vi "svc_Check for Resampled Signal Continuity (no state).vi"(0 "even angle signal":T5 {"even angle signal" format="%.2f"; "dr" format="%.2f"; "r0" format="%.2f"}, 1 "even angle channel info":T1={"channel name"="", "description"="", " channel info"={"sensor sensitivity"=1000.0, "engineering units"=1, "dB reference"=1.0, "custom label"="EU", "weighting filter"=0, "pregain"=0.0}} {"channel info"."pregain" format="%.2f"; "channel info"."weighting filter" items=["Linear", "A-weighting", "B-weighting", "C-weighting", "ITU-R 468-4", "Dolby", "CCITT", "C-message", "Wb", "Wc", "Wd", "We", "Wf", "Wh", "Wj", "Wk", "Wm", "AES17 20 kHz lowpass", "AES17 40 kHz lowpass", "AES17 20 kHz highpass", "AES17 40 kHz highpass"]; "channel info"."dB reference" format="%^.1e"; "channel info"."engineering units" items=["custom..."=0, "V"=1, "A"=21, "C"=30, "pC"=31, "s"=32, "-"=29, "Pa"=2, "N"=20, "g"=3, "m/s^2"=4, "m/s"=5, "m"=6, "mm/s"=12, "mm"=13, "micron/s"=14, "micron"=15, "in/s^2"=7, "in/s"=8, "in"=9, "mil/s"=10, "mil"=11, "rad/s^2"=16, "rad/s"=17, "rad"=18, "deg/s^2"=26, "deg/s"=27, "deg"=28, "RPM"=22, "cycle/s^2"=23, "Hz"=24, "cycle"=25, "strain"=19]; "channel info"."sensor sensitivity" format="%#_5f"}, 2 "parameter controls":T6, 5 "error in (no error)":errorcluster, 6 "reset":bool, 7 "expected even angle channel info":T1={"channel name"="", "description"="", " channel info"={"sensor sensitivity"=1000.0, "engineering units"=1, "dB reference"=1.0, "custom label"="EU", "weighting filter"=0, "pregain"=0.0}} {"channel info"."pregain" format="%.2f"; "channel info"."weighting filter" items=["Linear", "A-weighting", "B-weighting", "C-weighting", "ITU-R 468-4", "Dolby", "CCITT", "C-message", "Wb", "Wc", "Wd", "We", "Wf", "Wh", "Wj", "Wk", "Wm", "AES17 20 kHz lowpass", "AES17 40 kHz lowpass", "AES17 20 kHz highpass", "AES17 40 kHz highpass"]; "channel info"."dB reference" format="%^.1e"; "channel info"."engineering units" items=["custom..."=0, "V"=1, "A"=21, "C"=30, "pC"=31, "s"=32, "-"=29, "Pa"=2, "N"=20, "g"=3, "m/s^2"=4, "m/s"=5, "m"=6, "mm/s"=12, "mm"=13, "micron/s"=14, "micron"=15, "in/s^2"=7, "in/s"=8, "in"=9, "mil/s"=10, "mil"=11, "rad/s^2"=16, "rad/s"=17, "rad"=18, "deg/s^2"=26, "deg/s"=27, "deg"=28, "RPM"=22, "cycle/s^2"=23, "Hz"=24, "cycle"=25, "strain"=19]; "channel info"."sensor sensitivity" format="%#_5f"}, 9 "expected signal parameters":cluster{"r0":dbl, "dr":dbl, "array length":i32}) -> (11 "next expected signal parameters":cluster{"r0":dbl, "dr":dbl, "array length":i32}, 13 "even angle channel info":T1={"channel name"="", "description"="", " channel info"={"sensor sensitivity"=1000.0, "engineering units"=1, "dB reference"=1.0, "custom label"="EU", "weighting filter"=0, "pregain"=0.0}} {"channel info"."pregain" format="%.2f"; "channel info"."weighting filter" items=["Linear", "A-weighting", "B-weighting", "C-weighting", "ITU-R 468-4", "Dolby", "CCITT", "C-message", "Wb", "Wc", "Wd", "We", "Wf", "Wh", "Wj", "Wk", "Wm", "AES17 20 kHz lowpass", "AES17 40 kHz lowpass", "AES17 20 kHz highpass", "AES17 40 kHz highpass"]; "channel info"."dB reference" format="%^.1e"; "channel info"."engineering units" items=["custom..."=0, "V"=1, "A"=21, "C"=30, "pC"=31, "s"=32, "-"=29, "Pa"=2, "N"=20, "g"=3, "m/s^2"=4, "m/s"=5, "m"=6, "mm/s"=12, "mm"=13, "micron/s"=14, "micron"=15, "in/s^2"=7, "in/s"=8, "in"=9, "mil/s"=10, "mil"=11, "rad/s^2"=16, "rad/s"=17, "rad"=18, "deg/s^2"=26, "deg/s"=27, "deg"=28, "RPM"=22, "cycle/s^2"=23, "Hz"=24, "cycle"=25, "strain"=19]; "channel info"."sensor sensitivity" format="%#_5f"}, 14 "even angle signal":T5 {"even angle signal" format="%.2f"; "dr" format="%.2f"; "r0" format="%.2f"}, 15 "waveform parameter changed":bool, 16 "dt":dbl, 17 "array length":i32, 19 "error out":errorcluster)   [LabVIEW 2017]
uses:
  <vilib>/addons/_NISVFA/_Shared subVIs/Controls/svc_Resampled Channel Info.ctl
  <vilib>/addons/_NISVFA/_Shared subVIs/Controls/svc_Channel Info.ctl
  <vilib>/addons/_NISVFA/_Shared subVIs/Controls/svc_Engineering Units Text Ring.ctl
  <vilib>/addons/_NISVFA/_Shared subVIs/Controls/svc_Weighting Filter Text Ring.ctl
panel:
  in  "exact comparison for dr?":bool=TRUE
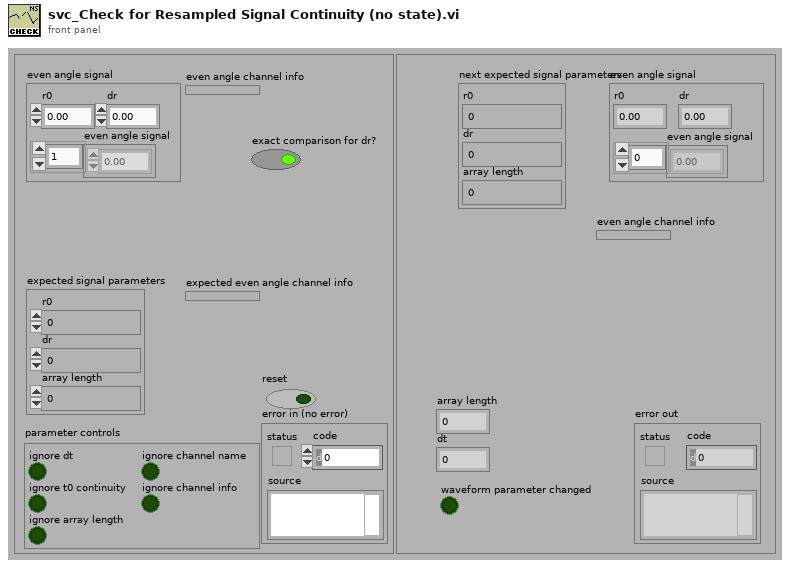
[diagram p1: front panel]
types:
  T1 = typedef "svc_Resampled Channel Info.ctl" = cluster{"channel name":string, "description":string, " channel info":T2}
  T2 = typedef "svc_Channel Info.ctl" = cluster{"sensor sensitivity":dbl, "engineering units":T3, "dB reference":dbl, "custom label":string, "weighting filter":T4, "pregain":dbl}
  T3 = typedef "svc_Engineering Units Text Ring.ctl" = u16
  T4 = typedef "svc_Weighting Filter Text Ring.ctl" = u16
  T5 = cluster{"r0":dbl, "dr":dbl, "even angle signal":dbl[]}
  T6 = cluster{"ignore dt":bool, "ignore t0 continuity":bool, "ignore array length":bool, "ignore channel info":bool, "ignore channel name":bool}
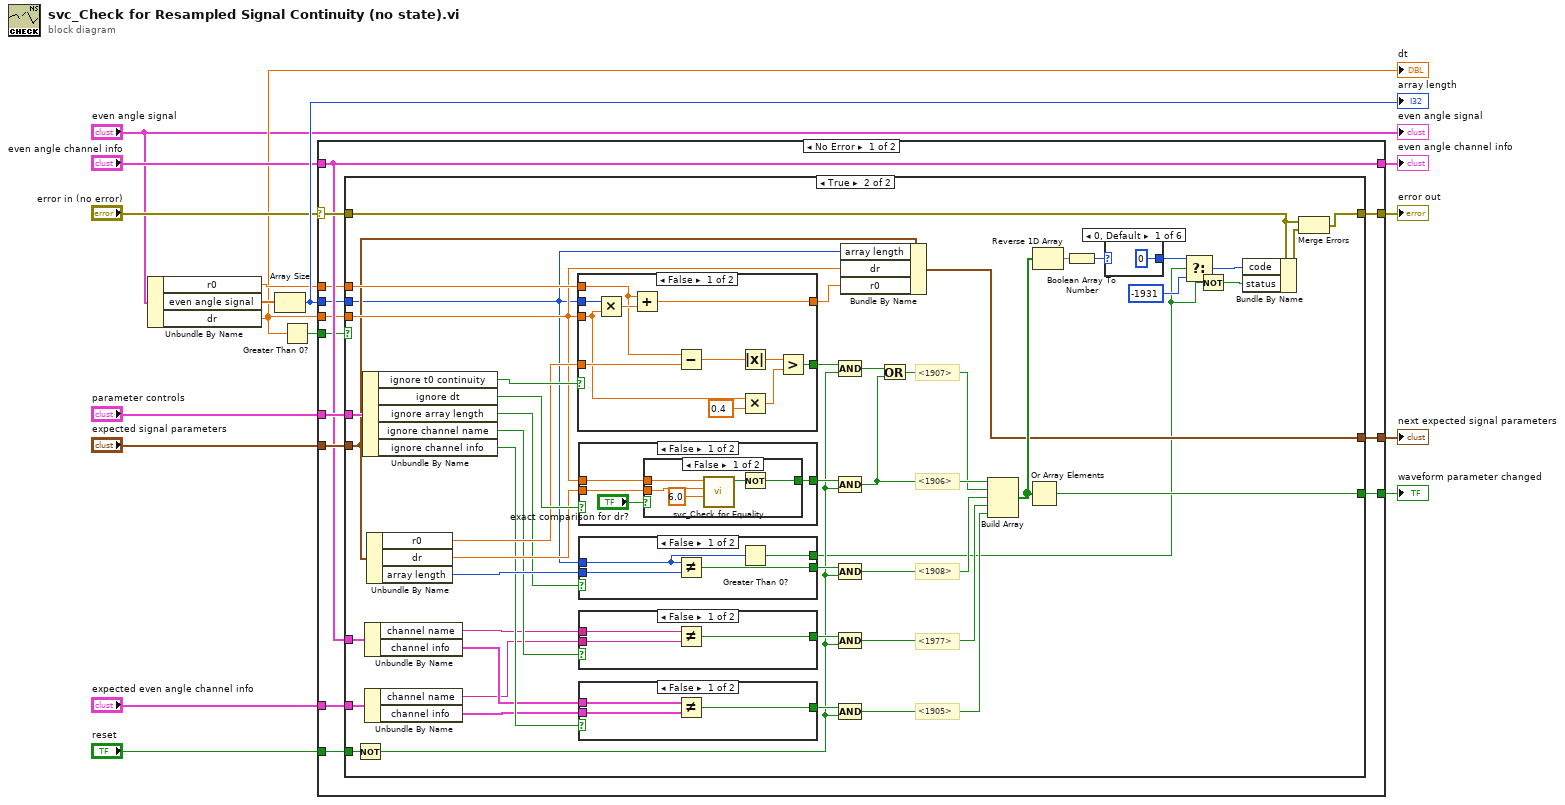
[diagram p0: block diagram]
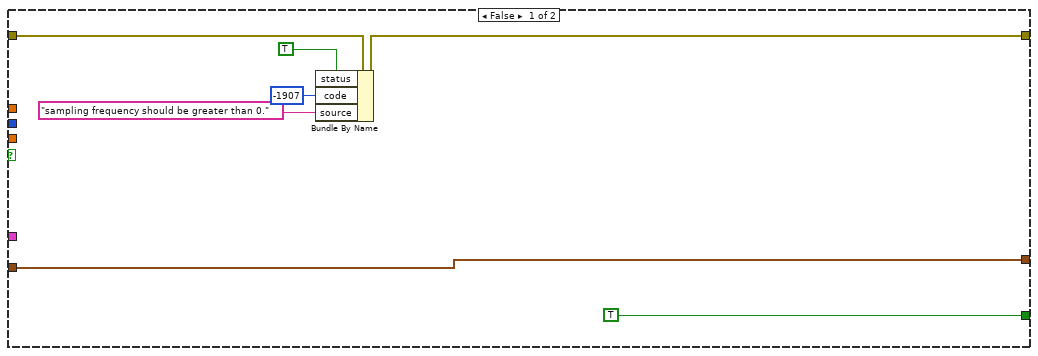
[diagram p2: hidden frame]
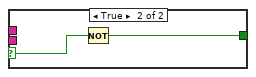
[diagram p3: hidden frame]
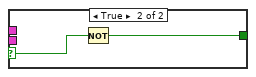
[diagram p4: hidden frame]
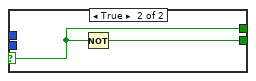
[diagram p5: hidden frame]
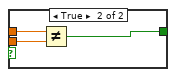
[diagram p6: hidden frame]
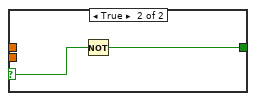
[diagram p7: hidden frame]
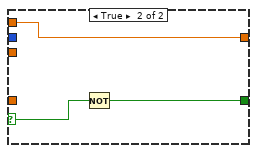
[diagram p8: hidden frame]
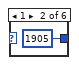
[diagram p9: hidden frame]
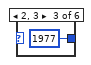
[diagram p10: hidden frame]
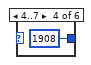
[diagram p11: hidden frame]
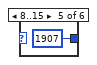
[diagram p12: hidden frame]
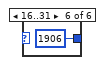
[diagram p13: hidden frame]
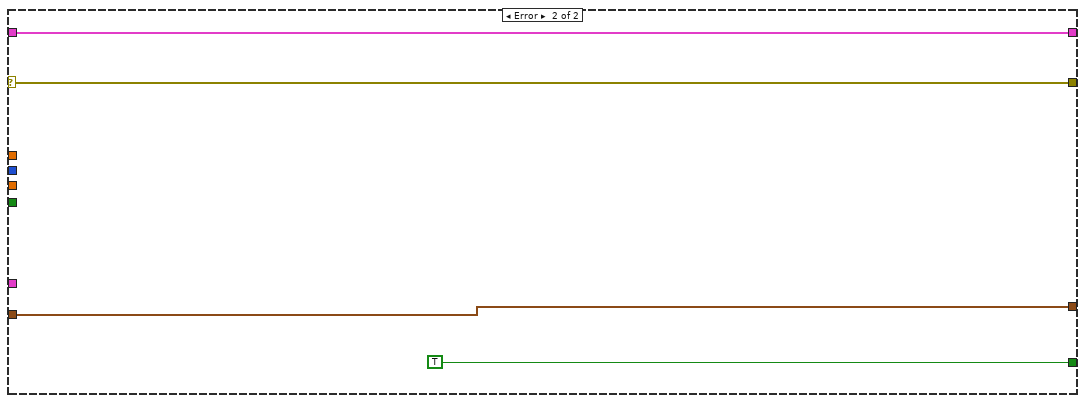
[diagram p14: hidden frame]
diagram:
  n1 = Unbundle By Name("even angle signal") -> ("r0"=w4:dbl, "even angle signal"=w3:dbl[], "dr"=w2:dbl)
  "dt" <- w2
  n2 = Array Size(array=w3) -> (size(s)=w7:i32)
  "array length" <- w7
  n3 = Greater Than 0?(x=w2) -> (x > 0?=w8:bool)
  n4 = case shown="No Error" "error in (no error)" {
    selector: "error in (no error)" -> [w29 w136]
    tunnel: [w28 w136] -> w16
    tunnel: "expected signal parameters" -> [w27 w133]
    tunnel: [w26 w133] -> w14
    tunnel: "parameter controls" -> [w25 _]
    tunnel: [w24 TRUE] -> w12
    tunnel: "reset" -> [w23 _]
    tunnel: "even angle channel info" -> [w21 w134]
    tunnel: "expected even angle channel info" -> [w22 _]
    tunnel: [w21 w134] -> w9
    tunnel: w4 -> [w20 _]
    tunnel: w7 -> [w19 _]
    tunnel: w2 -> [w18 _]
    tunnel: w8 -> [w17 _]
    frame No Error {
      n5 = case shown="True" w17 {
        tunnel: w29 -> [w35 w41]
        tunnel: [w31 w40] -> w28
        tunnel: w27 -> [w30 w57]
        tunnel: [w30 w58] -> w26
        tunnel: w25 -> [_ w68]
        tunnel: [TRUE w61] -> w24
        tunnel: w23 -> [_ w69]
        tunnel: w21 -> [_ w50]
        tunnel: w22 -> [_ w48]
        tunnel: w18 -> [_ w59]
        tunnel: w20 -> [_ w60]
        tunnel: w19 -> [_ w55]
        frame False {
          n6 = Bundle By Name(cluster=w35, "status"=TRUE, "code"=-1907, "source"="sampling frequency should be greater than 0.") -> (w31:errorcluster)
        }
        frame True {
          # "<1977>"
          # "<1906>"
          # "<1905>"
          # "<1907>"
          # "<1908>"
          n7 = Not(x=w69) -> (.not. x?=w53:bool)
          n8 = Unbundle By Name(w68) -> ("ignore t0 continuity"=w67:bool, "ignore dt"=w66:bool, "ignore array length"=w63:bool, "ignore channel name"=w51:bool, "ignore channel info"=w62:bool)
          n9 = Unbundle By Name(w50) -> ("channel name"=w45:string, "channel info"=w49:T2)
          n10 = Unbundle By Name(w48) -> ("channel name"=w46:string, "channel info"=w47:T2)
          n11 = Unbundle By Name(w57) -> ("r0"=w64:dbl, "dr"=w65:dbl, "array length"=w71:i32)
          n12 = case shown="False" w67 {
            selector: w67 -> [_ w126]
            tunnel: [w123 w125] -> w81
            tunnel: w64 -> [w119 _]
            tunnel: w60 -> [w118 w124]
            tunnel: w55 -> [w117 _]
            tunnel: w59 -> [w116 _]
            tunnel: [w113 w124] -> w56
            frame False {
              n13 = Multiply(x=w117, y=w116) -> (x*y=w122:dbl)
              n14 = Add(x=w118, y=w122) -> (x+y=w113:dbl)
              n15 = Subtract(x=w118, y=w119) -> (x-y=w114:dbl)
              n16 = Absolute Value(x=w114) -> (abs(x)=w115:dbl)
              n17 = Multiply(x=w116, y=0.4 ("x")) -> (x*y=w120:dbl)
              n18 = Greater?(x=w115, y=w120) -> (0:w123:bool)
            }
            frame True {
              n19 = Not(x=w126) -> (.not. x?=w125:bool)
            }
          }
          n20 = case shown="False" w66 {
            selector: w66 -> [_ w112]
            tunnel: [w102 w111] -> w82
            tunnel: w65 -> [w101 _]
            tunnel: w59 -> [w100 _]
            frame False {
              n21 = case shown="False" "exact comparison for dr?" {
                tunnel: [w107 w108] -> w102
                tunnel: w101 -> [w103 w109]
                tunnel: w100 -> [w104 w110]
                frame False {
                  n22 = call <vilib>:"svc_Check for Equality.vi"("desired precision"=6.0, "n2"=w103, "n1"=w104) -> ("equal?"=w106:bool)  [unwired: 7 in, 1 out]
                  n23 = Not(x=w106) -> (.not. x?=w107:bool)
                }
                frame True {
                  n24 = Not Equal?(x=w110, y=w109) -> (x != y?=w108:bool)
                }
              }
            }
            frame True {
              n25 = Not(x=w112) -> (.not. x?=w111:bool)
            }
          }
          n26 = case shown="False" w63 {
            selector: w63 -> [_ w97]
            tunnel: w55 -> [w94 _]
            tunnel: [w96 w98] -> w80
            tunnel: w71 -> [w95 _]
            tunnel: [w93 w97] -> w39
            frame False {
              n27 = Not Equal?(x=w94, y=w95) -> (x != y?=w96:bool)
              n28 = Greater Than 0?(x=w94) -> (x > 0?=w93:bool)
            }
            frame True {
              n29 = Not(x=w97) -> (.not. x?=w98:bool)
            }
          }
          n30 = case shown="False" w51 {
            selector: w51 -> [_ w87]
            tunnel: [w85 w86] -> w54
            tunnel: w46 -> [w84 _]
            tunnel: w45 -> [w83 _]
            frame False {
              n31 = Not Equal?(x=w83, y=w84) -> (x != y?=w85:bool)
            }
            frame True {
              n32 = Not(x=w87) -> (.not. x?=w86:bool)
            }
          }
          n33 = case shown="False" w62 {
            selector: w62 -> [_ w92]
            tunnel: [w90 w91] -> w79
            tunnel: w47 -> [w89 _]
            tunnel: w49 -> [w88 _]
            frame False {
              n34 = Not Equal?(x=w88, y=w89) -> (x != y?=w90:bool)
            }
            frame True {
              n35 = Not(x=w92) -> (.not. x?=w91:bool)
            }
          }
          n36 = Compound Arithmetic op=AND(w81, w53) -> (w78:bool)
          n37 = Compound Arithmetic op=AND(w82, w53) -> (w77:bool)
          n38 = Compound Arithmetic op=AND(w80, w53) -> (w74:bool)
          n39 = Compound Arithmetic op=AND(w54, w53) -> (w52:bool)
          n40 = Compound Arithmetic op=AND(w79, w53) -> (w75:bool)
          n41 = Bundle By Name(cluster=w57, "array length"=w55, "dr"=w59, "r0"=w56) -> (w58:cluster{"r0":dbl, "dr":dbl, "array length":i32})
          n42 = Or(x=w78, y=w77) -> (x .or. y?=w76:bool)
          n43 = Build Array(w77, w76, w74, w52, w75) -> (w70:bool[])
          n44 = Or Array Elements(Boolean array=w70) -> (logical OR=w61:bool)
          n45 = Reverse 1D Array(array=w70) -> (reversed array=w72:bool[])
          n46 = Boolean Array To Number(Boolean array=w72) -> (number=w73:u32)
          n47 = case shown="0, Default" w73 {
            tunnel: [0 ("code") 1905 ("code") 1977 ("code") 1908 ("code") 1907 ("code") 1906 ("code")] -> w44
            frame 0, Default {
            }
            frame 1 {
            }
            frame 2, 3 {
            }
            frame 4..7 {
            }
            frame 8..15 {
            }
            frame 16..31 {
            }
          }
          n48 = Select(t=w44, s=w39, f=-1931 ("t")) -> (s? t:f=w38:i32)
          n49 = Not(x=w39) -> (.not. x?=w42:bool)
          n50 = Bundle By Name(cluster=w41, "code"=w38, "status"=w42) -> (w37:errorcluster)
          n51 = Merge Errors(w41, w37) -> (w40:errorcluster)
        }
      }
    }
    frame Error {
    }
  }
  "error out" <- w16
  "next expected signal parameters" <- w14
  "waveform parameter changed" <- w12
  "even angle channel info" <- w9
  "even angle signal" <- "even angle signal"
